vi "GUI.ConfigureUI.vi"(8 "error in (no error)":errorcluster) -> (0 "error out":errorcluster, 1 "Log Path out":path, 2 "Canceled?":bool, 3 "gRPC Info":T4)   [LabVIEW 2025, in "XNET Bus Monitor Client.lvlib"]
uses:
  XNET Bus Monitor Client.lvlib
  Types/gRPC.ConnectionInfo.ctl
  <vilib>/gRPC/LabVIEW gRPC Library/Shared/grpcId.ctl
  xnet_can_bus_monitor_api_client/RPC Messages/ni_xnet_can_bm_api_CanMode.ctl
  xnet_can_bus_monitor_api_client/RPC Messages/ni_xnet_can_bm_api_FdIsoMode.ctl
  xnet_can_bus_monitor_api_client/RPC Messages/ni_xnet_can_bm_api_Termination.ctl
  xnet_can_bus_monitor_api_client/RPC Messages/ni_xnet_can_bm_api_InitializeSettingsRequest.ctl
  xnet_can_bus_monitor_api_client/RPC Messages/ni_xnet_can_bm_api_ConnectSettings.ctl
  xnet_can_bus_monitor_api_client/xnet_can_bus_monitor_api_client.lvlib
  <vilib>/gRPC/LabVIEW gRPC Library/grpc-lvsupport-release.lvlib
panel:
  in  "Log Folder Path":path
  in  "FD Baud_Rate":u64 format="%.0x"
  in  "Baud Rate":u64
  in  "Termination":T1
  in  "FD ISO Mode":T2
  in  "CAN Mode":T3
  in  "Cancel":bool
  in  "Connect":bool
  out "Found Port":u64
  in  "Check Connection":bool
  in  "Service Name":string
  in  "IP Address":string
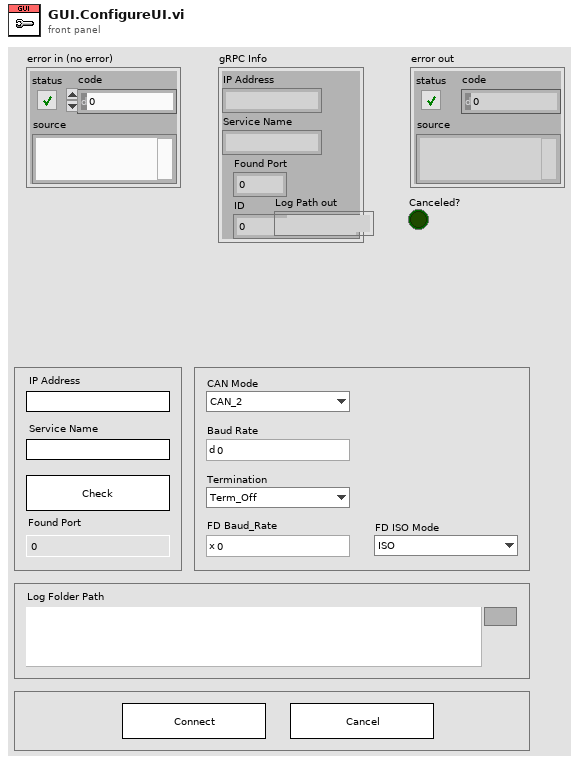
[diagram p1: front panel]
types:
  T1 = typedef "xnet_can_bus_monitor_api_client.lvlib/ni_xnet_can_bm_api_Termination.ctl" = enum32{"Term_Off", "Term_On"}
  T2 = typedef "xnet_can_bus_monitor_api_client.lvlib/ni_xnet_can_bm_api_FdIsoMode.ctl" = enum32{"ISO", "Non_ISO", "ISO_Legacy"}
  T3 = typedef "xnet_can_bus_monitor_api_client.lvlib/ni_xnet_can_bm_api_CanMode.ctl" = enum32{"CAN_2", "CAN_FD", "CAN_FD_BRS"}
  T4 = typedef "XNET Bus Monitor Client.lvlib/gRPC.ConnectionInfo.ctl" = cluster{"IP Address":string, "Service Name":string, "Found Port":u64, "ID":T5}
  T5 = typedef "grpc-lvsupport-release.lvlib/grpcId.ctl" = u64
  T6 = enum8{"Enabled", "Disabled", "Disabled and Grayed Out"}
  T7 = typedef "xnet_can_bus_monitor_api_client.lvlib/ni_xnet_can_bm_api_InitializeSettingsRequest.ctl" = cluster{"name":string, "connect_settings":T8, "default_filter_ids":u32[]}
  T8 = typedef "xnet_can_bus_monitor_api_client.lvlib/ni_xnet_can_bm_api_ConnectSettings.ctl" = cluster{"port":string, "can_mode":T3, "termination":T1, "baud_rate":u64, "fd_baud_rate":u64, "fd_iso_mode":T2}
  T9 = typedef "xnet_can_bus_monitor_api_client.lvlib/ni_xnet_can_bm_api_InitializeSettingsReply.ctl" = cluster{"error":T10}
  T10 = typedef "xnet_can_bus_monitor_api_client.lvlib/ni_xnet_can_bm_api_ErrorInfo.ctl" = errorcluster
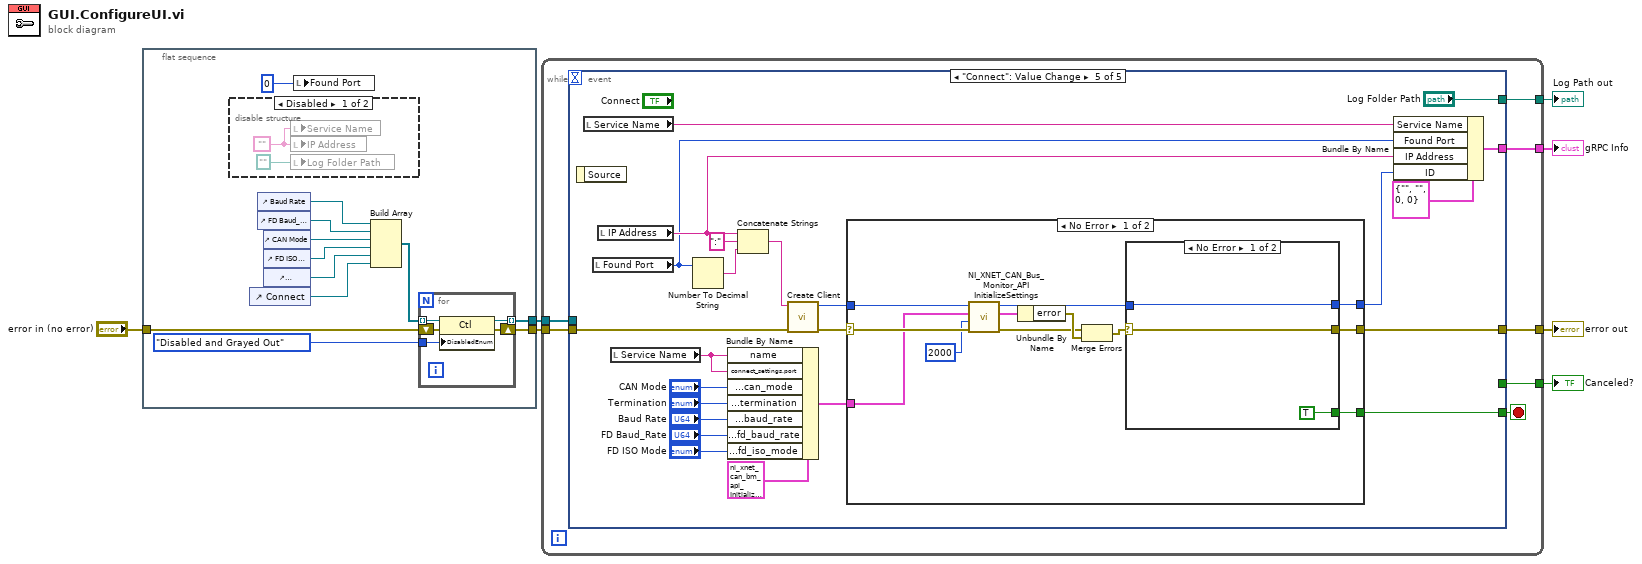
[diagram p0: block diagram]
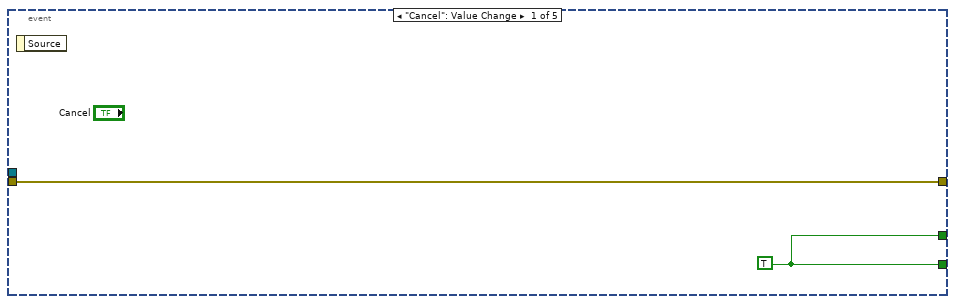
[diagram p3: hidden frame]
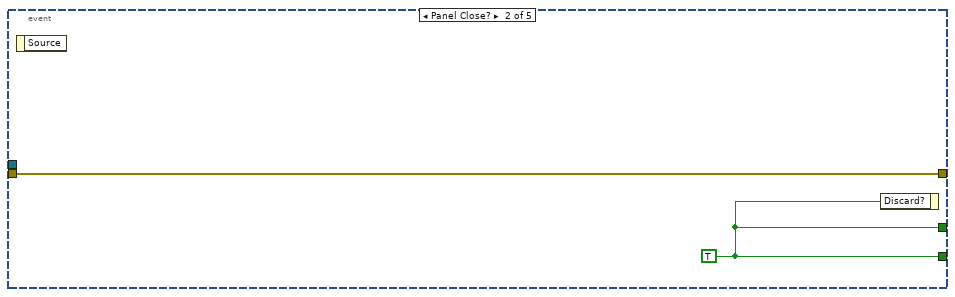
[diagram p4: hidden frame]
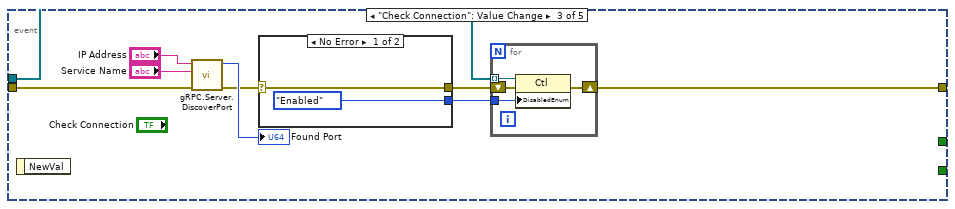
[diagram p5: hidden frame]
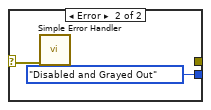
[diagram p6: hidden frame]
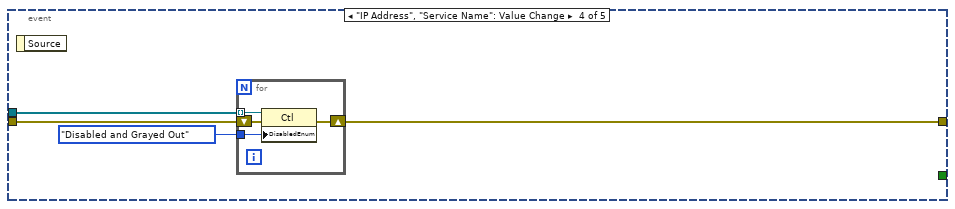
[diagram p7: hidden frame]
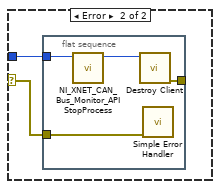
[diagram p8: hidden frame]
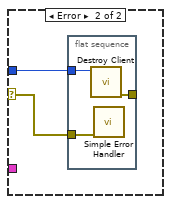
[diagram p9: hidden frame]
diagram:
  n1 = flat-sequence {
    tunnel: [w18] -> w6
    tunnel: [w17] -> w5
    tunnel: "error in (no error)" -> [w15]
    frame #0 {
      n2 = disable-structure shown="Disabled" {
        frame Disabled {
          w21 = ""
          n3 = local write "Service Name"(w21) -> ()
          n4 = local write "IP Address"(w21) -> ()
          n5 = local write "Log Folder Path"(path "") -> ()
        }
        frame Enabled {
        }
      }
      n6 = control-ref of="Connect"() -> (w9:refnum<vi>)
      n7 = control-ref of="Baud Rate"() -> (w14:refnum<vi>)
      n8 = control-ref of="FD Baud_Rate"() -> (w13:refnum<vi>)
      n9 = control-ref of="CAN Mode"() -> (w12:refnum<vi>)
      n10 = control-ref of="FD ISO Mode"() -> (w11:refnum<vi>)
      n11 = control-ref of="Termination"() -> (w10:refnum<vi>)
      n12 = local write "Found Port"(u64 0 ("Found Port")) -> ()
      n13 = Build Array(w14, w13, w12, w11, w10, w9) -> (w8:refnum<vi>[])
      n14 = for {
        tunnel: T6."Disabled and Grayed Out" ("Disabled") -> [w26]
        tunnel: [w25] -> w18 mode=indexing
        shift-right: [w24] -> w17
        shift-left: w15 -> [w23]
        tunnel: w8 -> [w22] mode=indexing
        n15 = property class="Ctl"(reference=w22, error in=w23, "DisabledEnum"=w26) -> (reference out=w25:refnum<vi>, error out=w24:errorcluster)
      }
    }
  }
  n16 = while {
    tunnel: [w32] -> w7
    tunnel: w6 -> [w31]
    tunnel: w5 -> [w30]
    tunnel: [w29] -> w3
    tunnel: [w28] -> w4
    tunnel: [w27] -> w1
    stop <- w33 stop-if-true
    n17 = event shown="[4] \"Connect\": Value Change" {
      selector: _ -> [_ _ _ _ _]
      dyn-events: _ -> [_ _ _ _ _]
      timeout: _ -> [_ _ _ _ _]
      tunnel: [w35 w37 _ _ w80] -> w33
      tunnel: [w35 w37 _ _ _] -> w32
      tunnel: w31 -> [_ _ w41 w57 _]
      tunnel: w30 -> [w34 w36 w44 w56 w82]
      tunnel: [w34 w36 w38 w55 w79] -> w29
      tunnel: [_ _ _ _ w77] -> w28
      tunnel: [_ _ _ _ "Log Folder Path"] -> w27
      event "Cancel": Value Change {
        w35 = TRUE
        n18 = event-data() -> ()  [unwired: 1 in, 1 out]
      }
      event Panel Close? {
        w37 = TRUE
        n19 = event-data() -> ()  [unwired: 1 in, 1 out]
        n20 = event-data("Discard?"=w37) -> ()  [unwired: 1 in, 1 out]
      }
      event "Check Connection": Value Change {
        n21 = event-data() -> ()  [unwired: 1 in, 1 out]
        n22 = call "gRPC.Server.DiscoverPort.vi"("error in (no error)"=w44, "Name"="Service Name", "IP Address"="IP Address") -> ("error out"=w42:errorcluster, "Port"=→"Found Port":i32)  [unwired: 7 in]
        n23 = case shown="No Error" w42 {
          selector: w42 -> [w52 w53]
          tunnel: [w52 _] -> w40
          tunnel: [T6."Enabled" ("Disabled") T6."Disabled and Grayed Out" ("Disabled")] -> w39
          frame No Error {
          }
          frame Error {
            n24 = call <vilib>:"Simple Error Handler.vi"("error in (no error)"=w53) -> ()  [unwired: 4 in, 5 out]
          }
        }
        n25 = for {
          tunnel: w41 -> [w50] mode=indexing
          tunnel: w39 -> [w48]
          shift-right: [w47] -> w38
          shift-left: w40 -> [w49]
          n26 = property class="Ctl"(reference=w50, error in=w49, "DisabledEnum"=w48) -> (error out=w47:errorcluster)  [unwired: 1 out]
        }
      }
      event "IP Address", "Service Name": Value Change {
        n27 = event-data() -> ()  [unwired: 1 in, 1 out]
        n28 = for {
          tunnel: T6."Disabled and Grayed Out" ("Disabled") -> [w62]
          tunnel: w57 -> [w61] mode=indexing
          shift-right: [w59] -> w55
          shift-left: w56 -> [w60]
          n29 = property class="Ctl"(reference=w61, error in=w60, "DisabledEnum"=w62) -> (error out=w59:errorcluster)  [unwired: 1 out]
        }
      }
      event "Connect": Value Change {
        n30 = event-data() -> ()  [unwired: 1 in, 1 out]
        n31 = local read "Service Name"() -> (w66:string)
        n32 = local read "Found Port"() -> (w75:u64)
        n33 = local read "IP Address"() -> (w78:string)
        n34 = local read "Service Name"() -> (w63:string)
        n35 = Number To Decimal String(number=w75) -> (decimal integer string=w84:string)  [unwired: 1 in]
        n36 = Bundle By Name(cluster=T7 {"name"="", "connect_settings"={"port"="", "can_mode"=enum."CAN_2", "termination"=enum."Term_Off", "baud_rate"=0, "fd_baud_rate"=0, "fd_iso_mode"=enum."ISO"}, "default_filter_ids"=[]} ("Request Data"), "name"=w63, "connect_settings.port"=w63, "connect_settings.can_mode"="CAN Mode", "connect_settings.termination"="Termination", "connect_settings.baud_rate"="Baud Rate", "connect_settings.fd_baud_rate"="FD Baud_Rate", "connect_settings.fd_iso_mode"="FD ISO Mode") -> (w67:T7)
        n37 = Concatenate Strings(w78, ":" ("string"), w84) -> (w83:string)
        n38 = call "Create Client.vi"("error in"=w82, "address"=w83) -> ("error out"=w81:errorcluster, "gRPC ID Out"=w74:T5)  [unwired: 8 in]
        n39 = case shown="No Error" w81 {
          selector: w81 -> [w96 w108]
          tunnel: [w97 _] -> w80
          tunnel: [w92 _] -> w79
          tunnel: w74 -> [w94 w107]
          tunnel: w67 -> [w87 _]
          tunnel: [w86 _] -> w65
          frame No Error {
            n40 = call "NI_XNET_CAN_Bus_Monitor_API InitializeSettings.vi"("error in"=w96, "timeout (ms)"=2000, "Request Data"=w87, "gRPC ID"=w94) -> ("error out"=w89:errorcluster, "Response Data"=w91:T9, "gRPC ID out"=w93:T5)  [unwired: 5 in]
            n41 = Unbundle By Name(w91) -> ("error"=w90:T10)
            n42 = Merge Errors(w89, w90) -> (w88:errorcluster)
            n43 = case shown="No Error" w88 {
              selector: w88 -> [w99 w102]
              tunnel: [TRUE _] -> w97
              tunnel: w93 -> [w98 w101]
              tunnel: [w99 _] -> w92
              tunnel: [w98 _] -> w86
              frame No Error {
              }
              frame Error {
                n44 = flat-sequence {
                  tunnel: w102 -> [w106]
                  tunnel: w101 -> [w103]
                  tunnel: [w105] -> _
                  frame #0 {
                    n45 = call "NI_XNET_CAN_Bus_Monitor_API StopProcess.vi"("gRPC ID"=w103) -> ("gRPC ID out"=w104:T5)  [unwired: 8 in, 2 out]
                    n46 = call "Destroy Client.vi"("gRPC ID"=w104) -> ("error out"=w105:errorcluster)  [unwired: 10 in]
                    n47 = call <vilib>:"Simple Error Handler.vi"("error in (no error)"=w106) -> ()  [unwired: 4 in, 5 out]
                  }
                }
              }
            }
          }
          frame Error {
            n48 = flat-sequence {
              tunnel: w108 -> [w111]
              tunnel: w107 -> [w110]
              tunnel: [w109] -> _
              frame #0 {
                n49 = call "Destroy Client.vi"("gRPC ID"=w110) -> ("error out"=w109:errorcluster)  [unwired: 10 in]
                n50 = call <vilib>:"Simple Error Handler.vi"("error in (no error)"=w111) -> ()  [unwired: 4 in, 5 out]
              }
            }
          }
        }
        n51 = Bundle By Name(cluster=T4 {"IP Address"="", "Service Name"="", "Found Port"=0, "ID"=0}, "Service Name"=w66, "Found Port"=w75, "IP Address"=w78, "ID"=w65) -> (w77:T4)
      }
    }
  }
  "Canceled?" <- w7
  "gRPC Info" <- w4
  "error out" <- w3
  "Log Path out" <- w1
